vi "ni579x Get Product ID.vi"(0 "Register Bus":refnum<class "ni579x Register Bus v1 Host.lvclass">=refnum, 11 "Error In":errorcluster) -> (4 "Register Bus (out)":refnum<class "ni579x Register Bus v1 Host.lvclass">, 6 "product ID":u16 format="%04x", 15 "Error Out":errorcluster)   [LabVIEW 2015]
uses:
  <instrlib>/ni579x/Register Bus/v1/Host/ni579x Register Bus v1 Host.lvclass
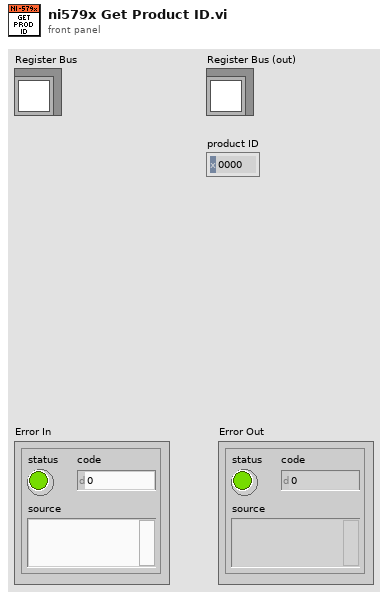
[diagram p1: front panel]
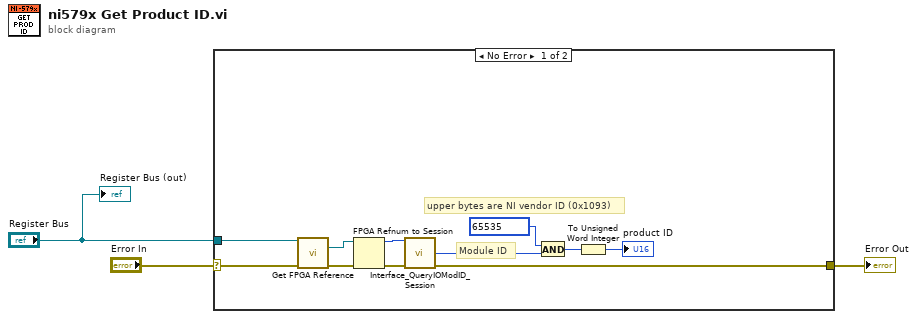
[diagram p0: block diagram]
diagram:
  n1 = case shown="No Error" "Error In" {
    selector: "Error In" -> [w14 w15]
    tunnel: [w9 w15] -> w2
    tunnel: "Register Bus" -> [w13 _]
    frame No Error {
      # "upper bytes are NI vendor ID (0x1093)"
      # "Module ID"
      n2 = call <instrlib>:"Get FPGA Reference.vi"("session in"=w13, "error in"=w14) -> ("fpga ref"=w8:refnum<k20>, "error out"=w12:errorcluster)  [unwired: 11 in, 1 out]
      n3 = FPGA Refnum to Session(4:w12, 7:w8) -> (0:w10:errorcluster, 3:w11:u64)
      n4 = call <vilib>:"Interface_QueryIOModID_Session.vi"("nifpga session"=w11, "error in"=w10) -> ("IO Module ID"=w7:u32, "error out"=w9:errorcluster)  [unwired: 11 in, 1 out]
      n5 = And(x=u32 65535, y=w7) -> (x .and. y?=w5:u32)
      n6 = To Unsigned Word Integer(number=w5) -> (unsigned 16bit integer=→"product ID":u16)
    }
    frame Error {
    }
  }
  "Error Out" <- w2
  "Register Bus (out)" <- "Register Bus"
